vi "DPD Configure.vi"(0 "RFmx Handle In":refnum<k21>, 1 "Selector String":string, 5 "DPD Configuration":T1={"Measurement Interval (s)"=0.0001, "DUT Average Input Power (dBm)"=-20.0, "Reference Waveform"={"x0"=0.0, "dx"=0.0, "y"=[]}, "Idle Duration Present"=0, "DPD Model"=0, "Threshold Enabled"=1, "Threshold Type"=0, "Threshold Level (dB or dBm)"=-20.0, "DPD LUT Type"=0, "Memory Polynomial Order"=3, "Memory Polynomial Memory Depth"=0, "Memory Polynomial Lead Order"=0, "Memory Polynomial Lead Memory Depth"=0, "Memory Polynomial Lag Order"=0, "Memory Polynomial Lag Memory Depth"=0, "Memory Polynomial Max Lag"=0, "Memory Polynomial Max Lead"=0, "Iterative DPD Enabled"=0, "Number of Iterations"=2} {"Number of Iterations" min=1; "Iterative DPD Enabled" items=["False", "True"]; "DPD LUT Type" items=["Log", "Linear"]; "Threshold Level (dB or dBm)" format="%.2f"; "Threshold Type" items=["Relative", "Absolute"]; "Threshold Enabled" items=["False", "True"]; "DPD Model" items=["Lookup Table", "Memory Polynomial", "Generalized Memory Polynomial"]; "Idle Duration Present" items=["False", "True"]; "Reference Waveform"."y" format="%.2f"; "Reference Waveform"."dx" format="%^.2e"; "Reference Waveform"."x0" format="%^.2e"; "DUT Average Input Power (dBm)" format="%.2f"; "Measurement Interval (s)" format="%.2p"}, 7 "DPD CFR Configuration":T2={"CFR Enabled"=0, "CFR Method"=0, "Max Iterations"=10, "Target PAPR Type"=0, "Target PAPR (dB)"=8.0, "Peak Windowing"={"Window Type"=7, "Window Length"=10}, "Sigmoid"={"Shaping Factor"=5.0, "Shaping Threshold (dB)"=-5.0}} {"Target PAPR Type" items=["Input PAPR", "Custom"]; "Peak Windowing"."Window Type" items=["Flat Top"=1, "Hanning"=2, "Hamming"=3, "Gaussian"=4, "Blackman"=5, "Blackman-Harris"=6, "Kaiser-Bessel"=7]; "CFR Method" items=["Clipping", "Peak Windowing", "Sigmoid"]; "CFR Enabled" items=["False", "True"]}, 11 "error in (no error)":errorcluster) -> (4 "RFmx Handle Out":refnum<k21>, 15 "error out":errorcluster)   [LabVIEW 2018, in "RFmxSpecAn.lvlib"]
uses:
  RFmxSpecAn.lvlib
  Typedefs/DPD Apply DPD CFR Configuration.ctl
  Typedefs/DPD Configuration.ctl
  <vilib>/RFmx/SpecAn/mx/RFmxSpecAn.llb/RFmxSpecAn Select Measurement (Single).vi
  <resource>/objmgr/RFmxSpecAn.rc
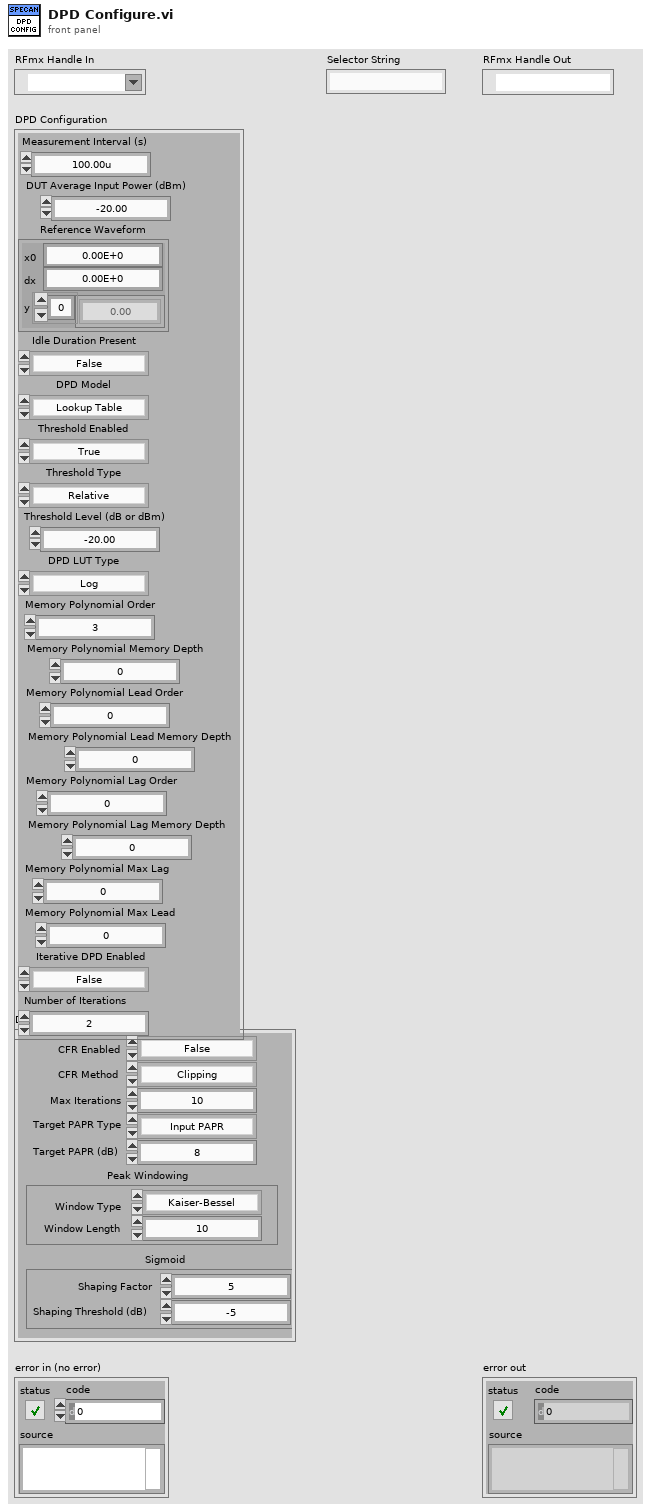
[diagram p1: front panel]
types:
  T1 = typedef "RFmxSpecAn.lvlib/DPD Configuration.ctl" = cluster{"Measurement Interval (s)":dbl, "DUT Average Input Power (dBm)":dbl, "Reference Waveform":cluster{"x0":dbl, "dx":dbl, "y":csg[]}, "Idle Duration Present":i32, "DPD Model":i32, "Threshold Enabled":i32, "Threshold Type":i32, "Threshold Level (dB or dBm)":dbl, "DPD LUT Type":i32, "Memory Polynomial Order":i32, "Memory Polynomial Memory Depth":i32, "Memory Polynomial Lead Order":i32, "Memory Polynomial Lead Memory Depth":i32, "Memory Polynomial Lag Order":i32, "Memory Polynomial Lag Memory Depth":i32, "Memory Polynomial Max Lag":i32, "Memory Polynomial Max Lead":i32, "Iterative DPD Enabled":i32, "Number of Iterations":i32}
  T2 = typedef "RFmxSpecAn.lvlib/DPD Apply DPD CFR Configuration.ctl" = cluster{"CFR Enabled":i32, "CFR Method":i32, "Max Iterations":i32, "Target PAPR Type":i32, "Target PAPR (dB)":dbl, "Peak Windowing":cluster{"Window Type":i32, "Window Length":i32}, "Sigmoid":cluster{"Shaping Factor":dbl, "Shaping Threshold (dB)":dbl}}
  T3 = enum16{"ACP", "CCDF", "CHP", "FCnt", "Harmonics", "OBW", "SEM", "Spectrum", "Spur", "TXP", "AMPM", "DPD", "IQ", "IM", "NF", "PhaseNoise"}
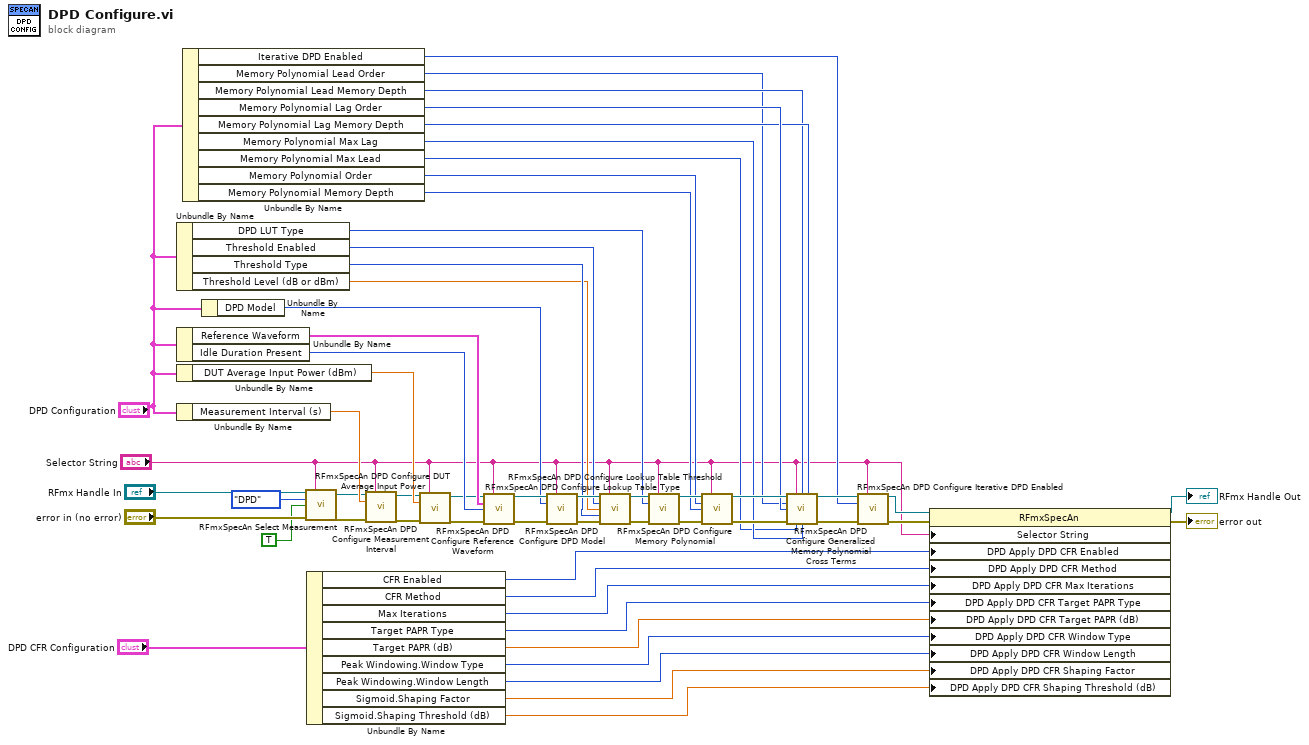
[diagram p0: block diagram]
diagram:
  n1 = Unbundle By Name("DPD Configuration") -> ("DPD LUT Type"=w28:i32, "Threshold Enabled"=w31:i32, "Threshold Type"=w30:i32, "Threshold Level (dB or dBm)"=w29:dbl)
  n2 = Unbundle By Name("DPD Configuration") -> ("Reference Waveform"=w51:cluster{"x0":dbl, "dx":dbl, "y":csg[]}, "Idle Duration Present"=w52:i32)
  n3 = Unbundle By Name("DPD Configuration") -> ("DUT Average Input Power (dBm)"=w50:dbl)
  n4 = Unbundle By Name("DPD Configuration") -> ("Measurement Interval (s)"=w49:dbl)
  n5 = Unbundle By Name("DPD Configuration") -> ("Iterative DPD Enabled"=w3:i32, "Memory Polynomial Lead Order"=w20:i32, "Memory Polynomial Lead Memory Depth"=w21:i32, "Memory Polynomial Lag Order"=w23:i32, "Memory Polynomial Lag Memory Depth"=w22:i32, "Memory Polynomial Max Lag"=w25:i32, "Memory Polynomial Max Lead"=w24:i32, "Memory Polynomial Order"=w27:i32, "Memory Polynomial Memory Depth"=w26:i32)
  n6 = Unbundle By Name("DPD Configuration") -> ("DPD Model"=w32:i32)
  n7 = call-poly <vilib>:"RFmxSpecAn Select Measurement.vi"("Instrument Handle In"="RFmx Handle In", "Selector String"="Selector String", "Measurement"=T3."DPD", "Enable All Traces"=TRUE, "error in (no error)"="error in (no error)") -> ("Instrument Handle Out"=w48:refnum<k21>, "error out"=w47:errorcluster)  [unwired: 9 in]
  n8 = Unbundle By Name("DPD CFR Configuration") -> ("CFR Enabled"=w11:i32, "CFR Method"=w19:i32, "Max Iterations"=w18:i32, "Target PAPR Type"=w17:i32, "Target PAPR (dB)"=w16:dbl, "Peak Windowing.Window Type"=w15:i32, "Peak Windowing.Window Length"=w14:i32, "Sigmoid.Shaping Factor"=w13:dbl, "Sigmoid.Shaping Threshold (dB)"=w12:dbl)
  n9 = call <vilib>:"RFmxSpecAn DPD Configure Measurement Interval.vi"("Instrument Handle In"=w48, "Selector String"="Selector String", "Measurement Interval (s)"=w49, "error in (no error)"=w47) -> ("Instrument Handle Out"=w46:refnum<k21>, "error out"=w45:errorcluster)  [unwired: 10 in]
  n10 = call <vilib>:"RFmxSpecAn DPD Configure DUT Average Input Power.vi"("Instrument Handle In"=w46, "Selector String"="Selector String", "DUT Average Input Power (dBm)"=w50, "error in (no error)"=w45) -> ("Instrument Handle Out"=w44:refnum<k21>, "error out"=w43:errorcluster)  [unwired: 10 in]
  n11 = call <vilib>:"RFmxSpecAn DPD Configure Reference Waveform.vi"("Instrument Handle In"=w44, "Selector String"="Selector String", "Reference Waveform"=w51, "Idle Duration Present"=w52, "error in (no error)"=w43) -> ("Instrument Handle Out"=w38:refnum<k21>, "error out"=w37:errorcluster)  [unwired: 9 in]
  n12 = call <vilib>:"RFmxSpecAn DPD Configure DPD Model.vi"("Instrument Handle In"=w38, "Selector String"="Selector String", "DPD Model"=w32, "error in (no error)"=w37) -> ("Instrument Handle Out"=w42:refnum<k21>, "error out"=w41:errorcluster)  [unwired: 10 in]
  n13 = call <vilib>:"RFmxSpecAn DPD Configure Lookup Table Threshold.vi"("Instrument Handle In"=w42, "Selector String"="Selector String", "Threshold Enabled"=w31, "Threshold Level (dB or dBm)"=w29, "Threshold Type"=w30, "error in (no error)"=w41) -> ("Instrument Handle Out"=w36:refnum<k21>, "error out"=w35:errorcluster)  [unwired: 8 in]
  n14 = call <vilib>:"RFmxSpecAn DPD Configure Lookup Table Type.vi"("Instrument Handle In"=w36, "Selector String"="Selector String", "DPD LUT Type"=w28, "error in (no error)"=w35) -> ("Instrument Handle Out"=w34:refnum<k21>, "error out"=w33:errorcluster)  [unwired: 10 in]
  n15 = call <vilib>:"RFmxSpecAn DPD Configure Memory Polynomial.vi"("Instrument Handle In"=w34, "Selector String"="Selector String", "Memory Polynomial Order"=w27, "Memory Polynomial Memory Depth"=w26, "error in (no error)"=w33) -> ("Instrument Handle Out"=w40:refnum<k21>, "error out"=w39:errorcluster)  [unwired: 9 in]
  n16 = call <vilib>:"RFmxSpecAn DPD Configure Generalized Memory Polynomial Cross Terms.vi"("Instrument Handle In"=w40, "Selector String"="Selector String", "Memory Polynomial Lead Memory Depth"=w21, "Memory Polynomial Lag Memory Depth"=w22, "Memory Polynomial Lead Order"=w20, "Memory Polynomial Lag Order"=w23, "error in (no error)"=w39, "Memory Polynomial Max Lead"=w24, "Memory Polynomial Max Lag"=w25) -> ("Instrument Handle Out"=w5:refnum<k21>, "error out"=w10:errorcluster)  [unwired: 5 in]
  n17 = call <vilib>:"RFmxSpecAn DPD Configure Iterative DPD Enabled.vi"("Instrument Handle In"=w5, "Selector String"="Selector String", "Iterative DPD Enabled"=w3, "error in (no error)"=w10) -> ("Instrument Handle Out"=w4:refnum<k21>, "error out"=w6:errorcluster)  [unwired: 10 in]
  n18 = property class="RFmxSpecAn"(reference=w4, error in=w6, "Selector String"="Selector String", "DPD Apply DPD CFR Enabled"=w11, "DPD Apply DPD CFR Method"=w19, "DPD Apply DPD CFR Max Iterations"=w18, "DPD Apply DPD CFR Target PAPR Type"=w17, "DPD Apply DPD CFR Target PAPR (dB)"=w16, "DPD Apply DPD CFR Window Type"=w15, "DPD Apply DPD CFR Window Length"=w14, "DPD Apply DPD CFR Shaping Factor"=w13, "DPD Apply DPD CFR Shaping Threshold (dB)"=w12) -> (reference out=→"RFmx Handle Out":refnum<k21>, error out=→"error out":errorcluster)
